vi "class_data.vi"() -> ()   [LabVIEW 2010, in "GenericDataCollection.lvclass"]
uses:
  GenericDataCollection.lvclass
panel:
  in  "latest instance":refnum<class "GenericDataCollection.lvclass">
  in  "update queue":string="data collection update queue"
  in  "image output queue":string="data collection output queue"
  in  "data request queue name":string="data collection request queue"
  in  "locked by":string
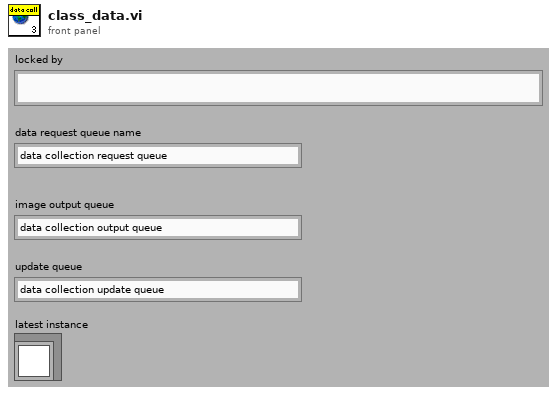
[diagram p1: front panel]
diagram:
